vi "Main.vi"() -> ()   [LabVIEW 2014, in "SquareBattle.lvclass"]
uses:
  SquareBattle.lvclass
  Runner/Runner.lvclass
  Runner Cluster.ctl
  Endigit Library/Endigit.lvlib
  Dashboard.ctl
panel:
  out "Start Battle":bool
  out "Total Squares":i32
  out "Intensity Graph 2":i32[][](graph)
  in  "Turn Update":u32=100
  in  "Exit":bool
  in  "UI Update":i32=100
  out "Dashboard":T1[](array[typedef])
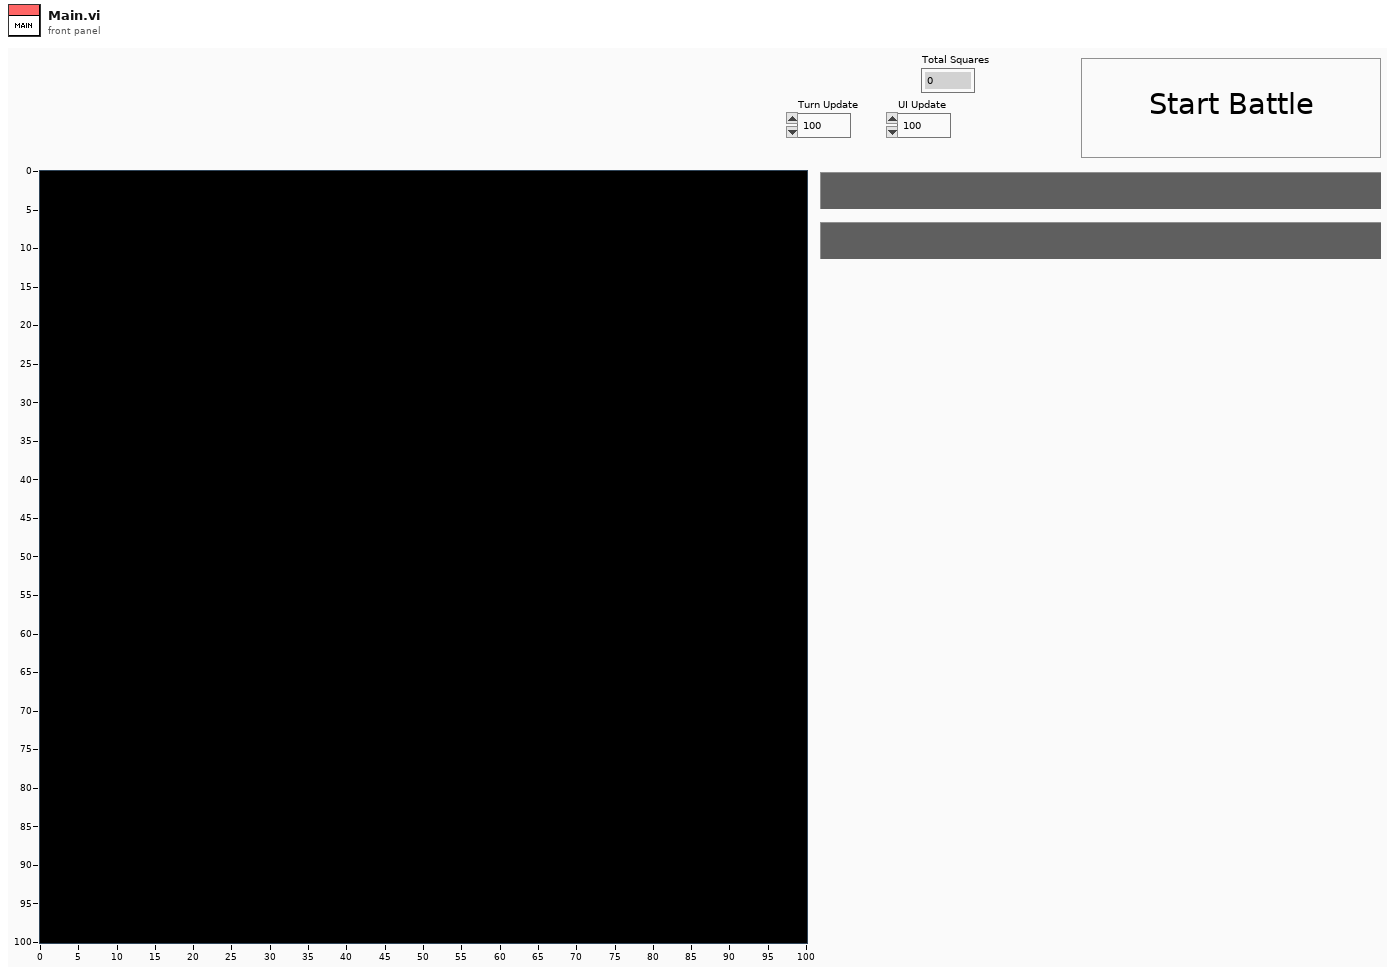
[diagram p1: front panel]
types:
  T1 = typedef "SquareBattle.lvclass/Dashboard.ctl" = cluster{"Color":u32, "Player":string, "Status":string}
  T2 = typedef "SquareBattle.lvclass/Runner Cluster.ctl" = cluster{"Alive?":bool, "RunnerRef":refnum<data-value>, "TeamIdx":i32, "Player #":i32, "NextPlay":u32}
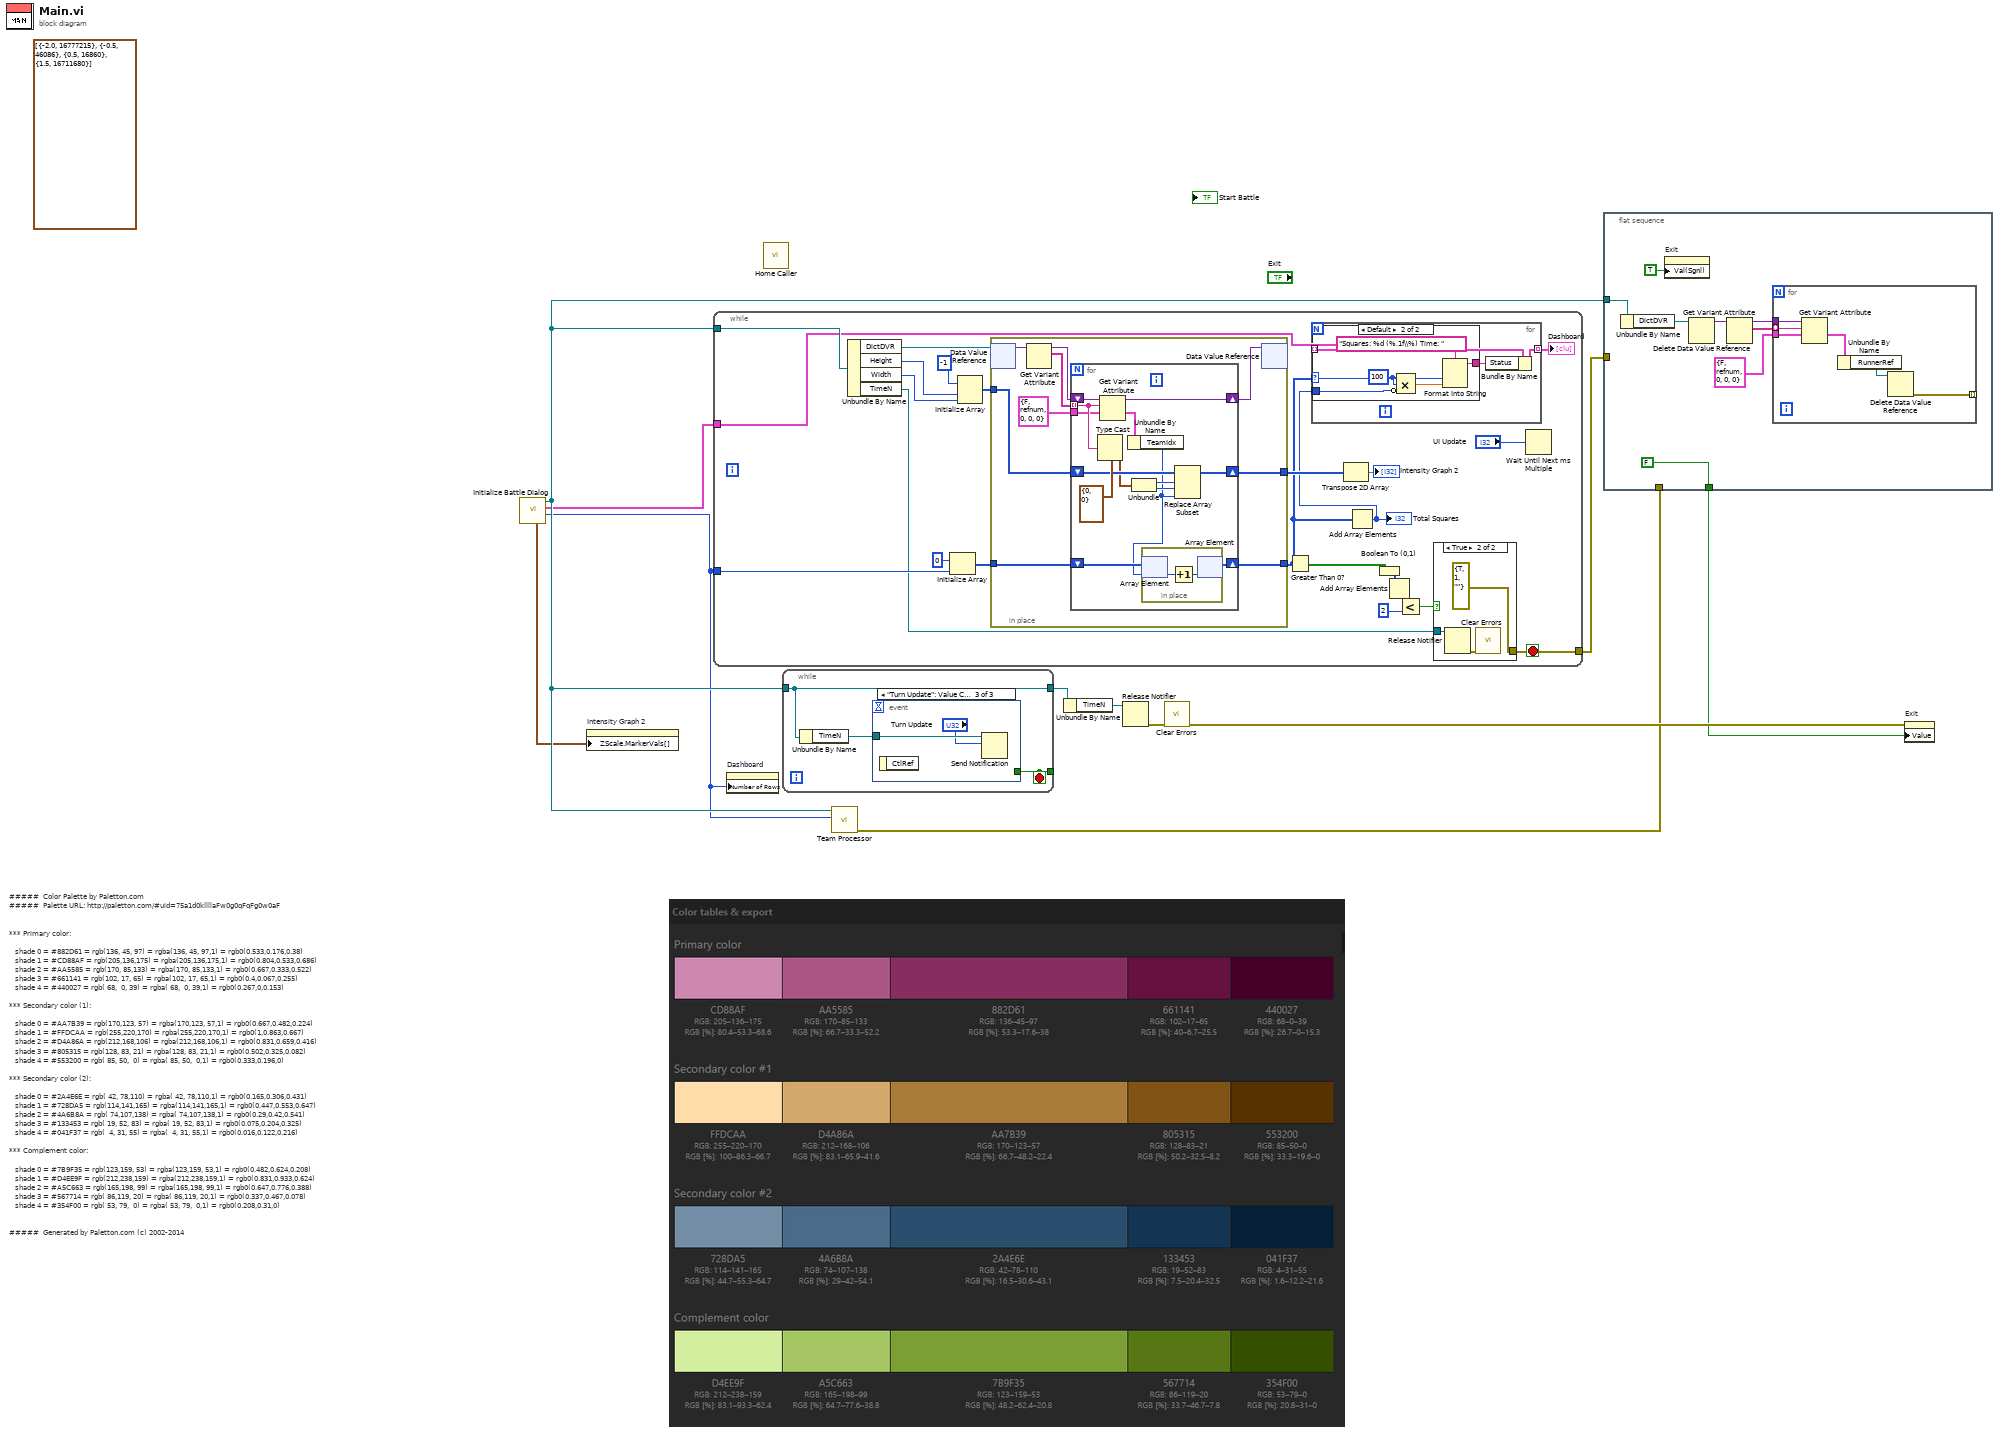
[diagram p0: block diagram]
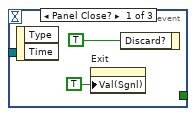
[diagram p2: hidden frame]
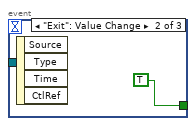
[diagram p3: hidden frame]
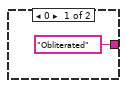
[diagram p4: hidden frame]
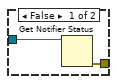
[diagram p5: hidden frame]
diagram:
  (unwired) cluster{dbl, u32}[] [{-2.0, 16777215}, {-0.5, 46086}, {0.5, 16860}, {1.5, 16711680}] ("Z Scale.Marker Values[]")
  # "#####  Color Palette by Paletton.com\n#####  Palette URL: http://paletton.com/#uid=75a1d0kllllaFw0g0qFqFg0w0aF\n\n\n*** Primary color:\n\n   shade 0 = #882D61 = rgb(136, 45, 97) = rgba(136, 45, 97,1) = rgb0(0.533,0.176,0.38)\n   shade 1 = #CD88AF = rgb(205,136,175) = rgba(205,136,175,1) = rgb0(0.804,0.533,0.686)\n   shade 2 = #AA5585 = rgb(170, 85,133) = rgba(170, 85,133,1) = rgb0(0.667,0.333,0.522)\n   shade 3 = #661141 = rgb(102, 17, 65) = rgba(102, 17, 65,1) = rgb0(0.4,0.067,0.255)\n   shade 4 = #440027 = rgb( 68,  0, 39) = rgba( 68,  0, 39,1) = rgb0(0.267,0,0.153)\n\n*** Secondary color (1):\n\n   shade 0 = #AA7B39 = rgb(170,123, 57) = rgba(170,123, 57,1) = rgb0(0.667,0.482,0.224)\n   shade 1 = #FFDCAA = rgb(255,220,170) = rgba(255,220,170,1) = rgb0(1,0.863,0.667)\n   shade 2 = #D4A86A = rgb(212,168,106) = rgba(212,168,106,1) = rgb0(0.831,0.659,0.416)\n   shade 3 = #805315 = rgb(128, 83, 21) = rgba(128, 83, 21,1) = rgb0(0.502,0.325,0.082)\n   shade 4 = #553200 = rgb( 85, 50,  0) = rgba( 85, 50,  0,1) = rgb0(0.333,0.196,0)\n\n*** Secondary color (2):\n\n   shade 0 = #2A4E6E = rgb( 42, 78,110) = rgba( 42, 78,110,1) = rgb0(0.165,0.306,0.431)\n   shade 1 = #728DA5 = rgb(114,141,165) = rgba(114,141,165,1) = rgb0(0.447,0.553,0.647)\n   shade 2 = #4A6B8A = rgb( 74,107,138) = rgba( 74,107,138,1) = rgb0(0.29,0.42,0.541)\n   shade 3 = #133453 = rgb( 19, 52, 83) = rgba( 19, 52, 83,1) = rgb0(0.075,0.204,0.325)\n   shade 4 = #041F37 = rgb(  4, 31, 55) = rgba(  4, 31, 55,1) = rgb0(0.016,0.122,0.216)\n\n*** Complement color:\n\n   shade 0 = #7B9F35 = rgb(123,159, 53) = rgba(123,159, 53,1) = rgb0(0.482,0.624,0.208)\n   shade 1 = #D4EE9F = rgb(212,238,159) = rgba(212,238,159,1) = rgb0(0.831,0.933,0.624)\n   shade 2 = #A5C663 = rgb(165,198, 99) = rgba(165,198, 99,1) = rgb0(0.647,0.776,0.388)\n   shade 3 = #567714 = rgb( 86,119, 20) = rgba( 86,119, 20,1) = rgb0(0.337,0.467,0.078)\n   shade 4 = #354F00 = rgb( 53, 79,  0) = rgba( 53, 79,  0,1) = rgb0(0.208,0.31,0)\n\n\n#####  Generated by Paletton.com (c) 2002-2014"
  n1 = call "Initialize Battle Dialog.vi"() -> ("# Players"=w1:i32, "Dashboard"=w2:T1[], "SquareBattle out"=w10:refnum<class "SquareBattle.lvclass">, "Intensity Graph Values"=w3:cluster{dbl, u32}[])  [unwired: 7 in, 1 out]
  n2 = property on="Intensity Graph 2" class="IntGraph (strict)"("ZScale.MarkerVals[]"=w3) -> ()  [unwired: 2 in, 2 out]
  n3 = while {
    tunnel: w10 -> [w34]
    tunnel: w1 -> [w24]
    tunnel: [w18] -> w8
    tunnel: w2 -> [w16]
    stop <- w18 stop-if-true
    n4 = Unbundle By Name(w34) -> ("DictDVR"=w33:refnum<data-value>, "Height"=w27:i32, "Width"=w26:i32, "TimeN"=w20:refnum<notifier>)
    n5 = Initialize Array(0 ("element"), w24) -> (w22:i32[])
    n6 = Initialize Array(-1, w27, w26) -> (w25:i32[][])
    n7 = in-place {
      in-place-border: [w60] -> w17
      in-place-border: w25 -> [w57]
      in-place-border: w22 -> [w53]
      in-place-border: [w52] -> w14
      n8 = in-place-dvr #1(w33) -> (w59:variant)  [unwired: 1 out]
      n9 = Get Variant Attribute(Variant=w59) -> (duplicate Variant=w56:variant, names=w58:string[])  [unwired: 3 in, 2 out]
      n10 = for {
        tunnel: w58 -> [w72] mode=indexing
        shift-right: [w68] -> w60
        shift-left: w57 -> [w69]
        shift-right: [w71] -> w55
        shift-left: w56 -> [w74]
        tunnel: T2 {"Alive?"=FALSE, "RunnerRef"=refnum, "TeamIdx"=0, "Player #"=0, "NextPlay"=0} ("Cluster") -> [w70]
        shift-right: [w63] -> w52
        shift-left: w53 -> [w62]
        n11 = Type Cast(type=cluster{"Y":i32, "X":i32} {"Y"=0, "X"=0}, x=w72) -> (*(type *) &x=w67:cluster{"Y":i32, "X":i32})
        n12 = Get Variant Attribute(Variant=w74, name=w72, default value (empty Variant)=w70) -> (duplicate Variant=w71:variant, value=w64:T2)  [unwired: 1 in, 2 out]
        n13 = Unbundle By Name(w64) -> ("TeamIdx"=w61:i32)
        n14 = Unbundle(w67) -> ("Y"=w66:i32, "X"=w65:i32)
        n15 = in-place {
          n16 = in-place-array #2(w62, w61) -> (w76:i32)
          n17 = Increment(x=w76) -> (x+1=w75:i32)
          n18 = in-place-array #2(w75) -> (w63:i32[])  [unwired: 1 out]
        }
        n19 = Replace Array Subset(array=w69, new element=w61, index (row)=w66, index (col)=w65) -> (w68:i32[][])
      }
      n20 = in-place-dvr #1(w55) -> ()  [unwired: 2 out]
    }
    n21 = Greater Than 0?(x=w14) -> (x > 0?=w32:bool[])
    n22 = Transpose 2D Array(2D array=w17) -> (transposed array=→"Intensity Graph 2":i32[][])
    n23 = Add Array Elements(numeric array=w14) -> (sum=w13:i32)
    "Total Squares" <- w13
    n24 = for {
      tunnel: w16 -> [w39] mode=indexing
      tunnel: [w38] -> w15 mode=indexing
      tunnel: w14 -> [w36] mode=indexing
      tunnel: w13 -> [w35]
      n25 = case shown="Default" w36 {
        selector: w36 -> [_ w43]
        tunnel: ["Obliterated" w45] -> w37
        tunnel: w35 -> [_ w42]
        frame 0 {
        }
        frame Default {
          n26 = Compound Arithmetic op=MULTIPLY(100 ("value"), w43, invert w42) -> (w44:dbl)
          n27 = Format Into String(format string="Squares: %d (%.1f\\%) Time: ", w43, w44) -> (resulting string=w45:string)  [unwired: 2 in, 1 out]
        }
      }
      n28 = Bundle By Name(cluster=w39, "Status"=w37) -> (w38:T1)
    }
    "Dashboard" <- w15
    n29 = Boolean To (0,1)(Boolean=w32) -> (0, 1=w31:i16[])
    n30 = Add Array Elements(numeric array=w31) -> (sum=w30:i16)
    n31 = Less?(x=w30, y=i16 2) -> (x < y?=w19:bool)
    n32 = case shown="True" w19 {
      tunnel: w20 -> [w48 w51]
      tunnel: [w47 errorcluster {"status"=TRUE, "code"=1, "source"=""} ("error out")] -> w18
      frame False {
        n33 = Get Notifier Status(notifier=w48) -> (error out=w47:errorcluster)  [unwired: 1 in, 4 out]
      }
      frame True {
        n34 = Release Notifier(notifier=w51) -> (error out=w49:errorcluster)  [unwired: 2 in, 2 out]
        n35 = call <vilib>:"Clear Errors.vi"("error in (no error)"=w49) -> ()  [unwired: 5 in, 2 out]
      }
    }
    n36 = Wait Until Next ms Multiple(millisecond multiple="UI Update") -> ()  [unwired: 1 out]
  }
  n37 = property on="Dashboard" class="Arr (strict)"("Number of Rows"=w1) -> ()  [unwired: 2 in, 2 out]
  n38 = call "Home Caller.vi"() -> ()  [unwired: 11 in]
  n39 = while {
    tunnel: w10 -> [w78]
    tunnel: [w78] -> w9
    tunnel: [w79] -> _
    stop <- w79 stop-if-true
    n40 = Unbundle By Name(w78) -> ("TimeN"=w77:refnum<notifier>)
    n41 = event shown="[2] \"Turn Update\": Value Change" {
      selector: _ -> [_ _ _]
      dyn-events: _ -> [_ _ _]
      timeout: _ -> [_ _ _]
      tunnel: [_ TRUE ("Discard?") _] -> w79
      tunnel: w77 -> [_ _ w84]
      event Panel Close? {
        n42 = event-data() -> ()  [unwired: 1 in, 2 out]
        n43 = property on="Exit" class="Bool (strict)"("Val(Sgnl)"=TRUE ("Value (Signaling)")) -> ()  [unwired: 2 in, 2 out]
        n44 = event-data("Discard?"=TRUE) -> ()  [unwired: 1 in, 1 out]
      }
      event "Exit": Value Change {
        n45 = event-data() -> ()  [unwired: 1 in, 4 out]
      }
      event "Turn Update": Value Change {
        n46 = event-data() -> ()  [unwired: 1 in, 1 out]
        n47 = Send Notification(notification="Turn Update", notifier=w84) -> ()  [unwired: 1 in, 2 out]
      }
    }
  }
  n48 = call "Team Processor.vi"("Team Count"=w1, "Maze 2.0.lvclass"=w10) -> ("error out"=w4:errorcluster)  [unwired: 9 in]
  n49 = Unbundle By Name(w9) -> ("TimeN"=w11:refnum<notifier>)
  n50 = Release Notifier(notifier=w11) -> (error out=w7:errorcluster)  [unwired: 2 in, 2 out]
  n51 = call <vilib>:"Clear Errors.vi"("error in (no error)"=w7) -> ("error out"=w6:errorcluster)  [unwired: 5 in, 1 out]
  n52 = flat-sequence {
    tunnel: w10 -> [w87]
    tunnel: w8 -> [_]
    tunnel: [FALSE ("Value (Signaling)")] -> w5
    tunnel: w4 -> [_]
    frame #0 {
      n53 = Unbundle By Name(w87) -> ("DictDVR"=w92:refnum<data-value>)
      n54 = property on="Exit" class="Bool (strict)"("Val(Sgnl)"=TRUE ("Value (Signaling)")) -> ()  [unwired: 2 in, 2 out]
      n55 = Delete Data Value Reference(data value reference=w92) -> (data value=w91:variant)  [unwired: 1 in, 1 out]
      n56 = Get Variant Attribute(Variant=w91) -> (duplicate Variant=w89:variant, names=w90:string[])  [unwired: 3 in, 2 out]
      n57 = for {
        tunnel: w90 -> [w97] mode=indexing
        tunnel: w89 -> [w98]
        tunnel: T2 {"Alive?"=FALSE, "RunnerRef"=refnum, "TeamIdx"=0, "Player #"=0, "NextPlay"=0} ("Cluster") -> [w96]
        tunnel: [w93] -> _ mode=indexing
        n58 = Get Variant Attribute(Variant=w98, name=w97, default value (empty Variant)=w96) -> (value=w95:T2)  [unwired: 1 in, 3 out]
        n59 = Unbundle By Name(w95) -> ("RunnerRef"=w94:refnum<data-value>)
        n60 = Delete Data Value Reference(data value reference=w94) -> (error out=w93:errorcluster)  [unwired: 1 in, 1 out]
      }
    }
  }
  n61 = property on="Exit" class="Bool (strict)"(error in=w6, "Value"=w5) -> ()  [unwired: 1 in, 2 out]
